vi "UnscentedKalmanFilter_Correct_B.vi"(11 "in UnscentedKalmanFiilter":T1) -> (3 "out UnscentedKalmanFiilter":T1)   [LabVIEW 2019, in "Trajectory_Library.lvlib"]
doc: "Creates a new LINEAR SYSTEM data cluster with the specified values. \n\n\nInputs: \n - XXX -- XXX.\n\nOutputs:\n - XXX -- XXX."
uses:
  UNSCENTED_KALMAN_FILTER.ctl
  <vilib>/Analysis/Matrix/Datatypes/RealMatrix.ctl
  MERWE_SCALED_SIGMA_PTS.ctl
  Trajectory_Library.lvlib
  <vilib>/Analysis/Matrix/NI_Matrix.lvlib
panel:
  # "State Estimate <Statess,1>"
  # "<States, States>"
  # "<States, ?>"
  # "<Statess,  States>"
  # "<Outputs, Outputs>"
  # "<?, 1>"
  # "<?, 1>"
  # "State Estimate <Statess,1>"
  # "<States, States>"
  # "<States, ?>"
  # "<Statess,  States>"
  # "<Outputs, Outputs>"
  # "<?, 1>"
  # "<?, 1>"
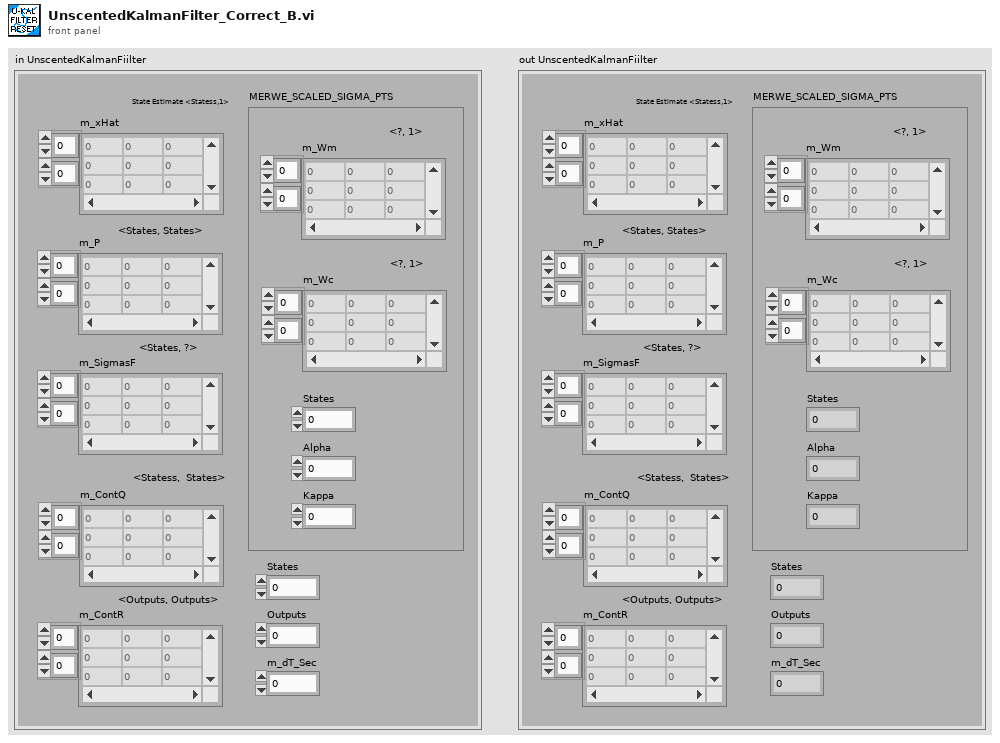
[diagram p1: front panel]
types:
  T1 = typedef "Trajectory_Library.lvlib/UNSCENTED_KALMAN_FILTER.ctl" = cluster{"m_P":T2, "m_xHat":T2, "States":i32, "Outputs":i32, "m_ContR":T2, "m_ContQ":T2, "m_SigmasF":T2, "m_dT_Sec":dbl, "MERWE_SCALED_SIGMA_PTS":T3}
  T2 = typedef "NI_Matrix.lvlib/RealMatrix.ctl" = dbl[][]
  T3 = typedef "Trajectory_Library.lvlib/MERWE_SCALED_SIGMA_PTS.ctl" = cluster{"m_Wm":T2, "States":i32, "Alpha":dbl, "m_Wc":T2, "Kappa":i32}
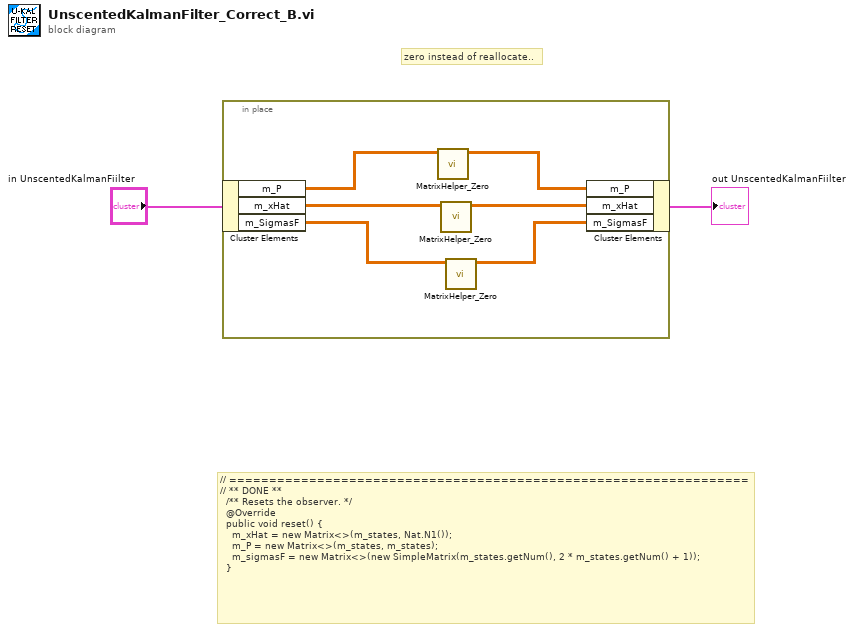
[diagram p0: block diagram]
diagram:
  # "zero instead of reallocate.."
  # "// =================================================================\n// ** DONE **\n  /** Resets the observer. */\n  @Override\n  public void reset() {\n    m_xHat = new Matrix<>(m_states, Nat.N1());\n    m_P = new Matrix<>(m_states, m_states);\n    m_sigmasF = new Matrix<>(new SimpleMatrix(m_states.getNum(), 2 * m_states.getNum() + 1));\n  }"
  n1 = in-place {
    n2 = in-place-cluster #1("in UnscentedKalmanFiilter") -> ("m_P"=w8:T2, "m_xHat"=w7:T2, "m_SigmasF"=w6:T2)
    n3 = call "MatrixHelper_Zero.vi"("input matrix"=w8) -> ("output matrix"=w5:T2)  [unwired: 10 in]
    n4 = call "MatrixHelper_Zero.vi"("input matrix"=w7) -> ("output matrix"=w4:T2)  [unwired: 10 in]
    n5 = call "MatrixHelper_Zero.vi"("input matrix"=w6) -> ("output matrix"=w3:T2)  [unwired: 10 in]
    n6 = in-place-cluster #1("m_P"=w5, "m_xHat"=w4, "m_SigmasF"=w3) -> (→"out UnscentedKalmanFiilter":T1)
  }
